vi "StringToVariant.vi"(7 "use system decimal point (T)":bool=TRUE, 11 "String-formatted Value":string) -> (2 "Value Class":T1, 3 "Variant-formatted Value":variant)   [LabVIEW 2013, in "CfgManager.Text.lvlib" / "Serializer.PlainText.lvclass"]
uses:
  Serializer.PlainText.lvclass
  Manager.Text/Character Class -- Enum.ctl
  Manager.Text/ConfigManager.Text.lvclass
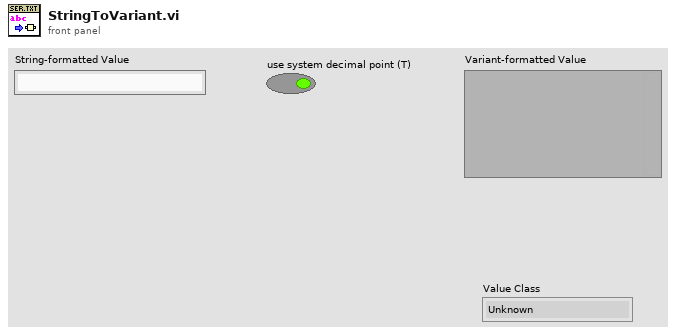
[diagram p1: front panel]
types:
  T1 = typedef "CfgManager.Text.lvlib/ConfigManager.Text.lvclass/Character Class -- Enum.ctl" = enum16{"Unknown", "Sign", "Zero", "Integer", "Float", "Complex", "Scientific", "Engineering", "Hexadecimal", "Binary", "Decimal", "Octal", "Unit", "Invalid", "Timestamp", "Boolean", "String", "Path", "null"}
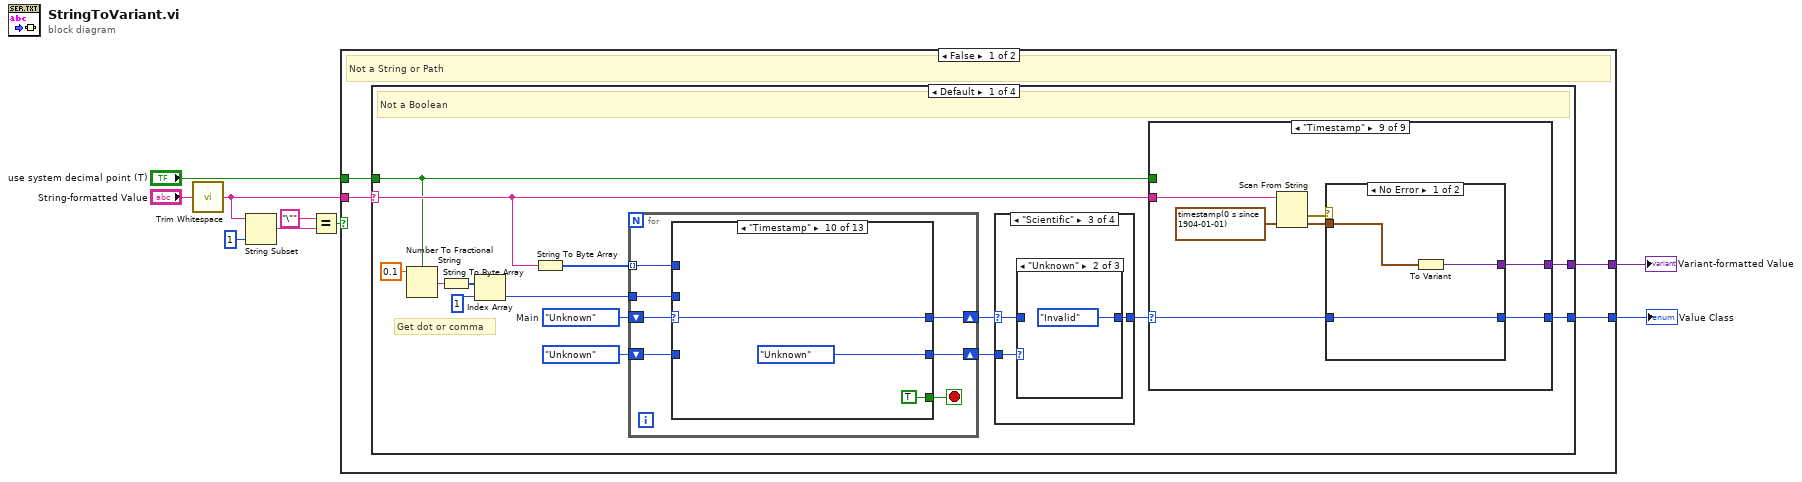
[diagram p0: block diagram]
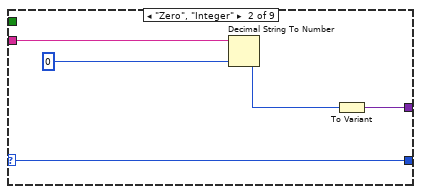
[diagram p3: hidden frame]
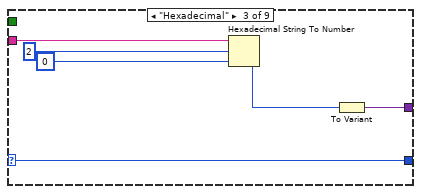
[diagram p4: hidden frame]
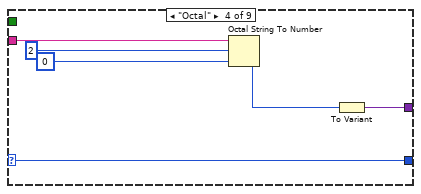
[diagram p5: hidden frame]
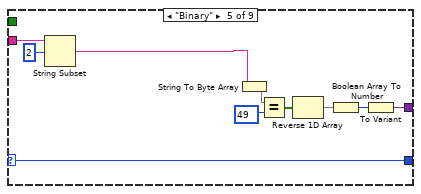
[diagram p6: hidden frame]
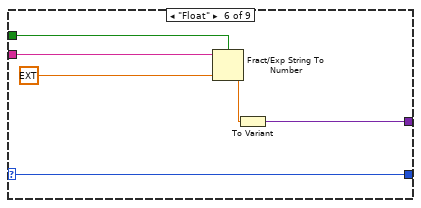
[diagram p7: hidden frame]
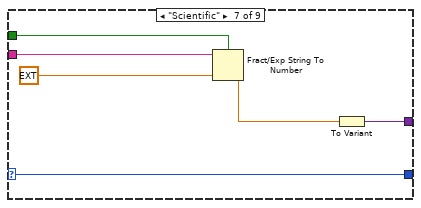
[diagram p8: hidden frame]
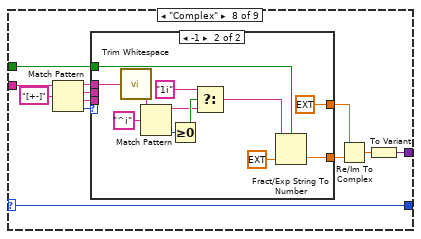
[diagram p9: hidden frame]
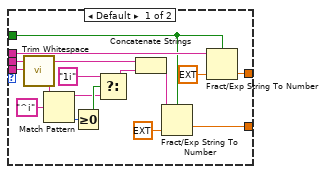
[diagram p10: hidden frame]
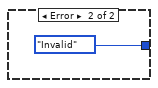
[diagram p11: hidden frame]
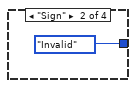
[diagram p13: hidden frame]
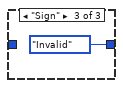
[diagram p15: hidden frame]
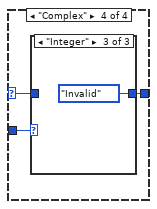
[diagram p16: hidden frame]
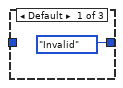
[diagram p17: hidden frame]
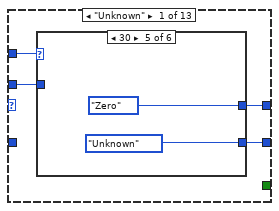
[diagram p19: hidden frame]
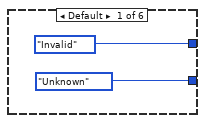
[diagram p20: hidden frame]
diagram:
  n1 = call <vilib>:"Trim Whitespace.vi"("string"="String-formatted Value") -> ("trimmed string"=w8:string)  [unwired: 1 in]
  n2 = String Subset(string=w8, length (rest)=1 ("length (rest)")) -> (substring=w6:string)  [unwired: 1 in]
  n3 = Equal?(x="\"", y=w6) -> (x = y?=w4:bool)
  n4 = case shown="False" w4 {
    tunnel: w8 -> [w13 w387]
    tunnel: [w12 w390] -> w9
    tunnel: [w11 w382] -> w3
    tunnel: "use system decimal point (T)" -> [w10 _]
    frame False {
      # "Not a String or Path"
      n5 = case shown="Default" w13 {
        selector: w13 -> [w23 _ _ _]
        tunnel: [w22 w374 w377 w381] -> w12
        tunnel: [w21 Character_Class_--_Enum."Boolean" Character_Class_--_Enum."Boolean" Character_Class_--_Enum."null"] -> w11
        tunnel: w10 -> [w18 _ _ _]
        frame Default {
          w27 = Character_Class_--_Enum."Unknown"  # Main
          # "Get dot or comma"
          # "Not a Boolean"
          n6 = Number To Fractional String(use system decimal point (T)=w18, number=0.1) -> (F-format string=w16:string)  [unwired: 2 in]
          n7 = String To Byte Array(string=w16) -> (unsigned byte array=w17:u8[])
          n8 = Index Array(array=w17, index=1 ("length (rest)")) -> (element=w14:u8)
          n9 = String To Byte Array(string=w23) -> (unsigned byte array=w28:u8[])
          n10 = for {
            tunnel: w28 -> [w139] mode=indexing
            shift-right: [w138] -> w26
            shift-left: w27 -> [w140]
            shift-right: [w136] -> w25
            shift-left: Character_Class_--_Enum."Unknown" -> [w137]
            tunnel: w14 -> [w134]
            stop <- w135 stop-if-true
            n11 = case shown="\"Timestamp\"" w140 {
              selector: w140 -> [_ w163 w167 w186 w217 w240 w246 w252 w258 w264 w267 w283 w324]
              tunnel: w139 -> [w144 _ w169 w188 w219 w242 w248 w254 w260 _ w269 w285 w326]
              tunnel: [w143 w163 w168 w187 w218 w241 w247 w253 w259 w264 w268 w284 w325] -> w138
              tunnel: w137 -> [_ w162 w164 _ _ _ _ _ _ _ _ w282 w323]
              tunnel: [w142 w162 w165 w185 w216 Character_Class_--_Enum."Unknown" Character_Class_--_Enum."Unknown" Character_Class_--_Enum."Unknown" Character_Class_--_Enum."Unknown" Character_Class_--_Enum."Unknown" w266 w281 w322] -> w136
              tunnel: [_ TRUE _ _ _ _ _ _ _ TRUE _ _ _] -> w135
              tunnel: w134 -> [w141 _ w166 w184 w215 _ _ _ _ _ _ _ w321]
              frame "Unknown" {
                n12 = case shown="30" w144 {
                  selector: w144 -> [_ _ _ w155 _ _]
                  tunnel: [Character_Class_--_Enum."Invalid" Character_Class_--_Enum."Sign" Character_Class_--_Enum."Integer" w151 Character_Class_--_Enum."Zero" w160] -> w143
                  tunnel: [Character_Class_--_Enum."Unknown" Character_Class_--_Enum."Unknown" Character_Class_--_Enum."Unknown" Character_Class_--_Enum."Unknown" Character_Class_--_Enum."Unknown" w160] -> w142
                  tunnel: w141 -> [_ _ _ w156 _ _]
                  frame Default {
                  }
                  frame 43, 45 {
                  }
                  frame 49..57 {
                  }
                  frame 44, 46 {
                    n13 = Equal?(x=w155, y=w156) -> (x = y?=w154:bool)
                    n14 = Select(t=Character_Class_--_Enum."Float", s=w154, f=Character_Class_--_Enum."Invalid") -> (s? t:f=w151:T1)
                  }
                  frame 48 {
                  }
                  frame 105 {
                    w160 = Character_Class_--_Enum."Complex"
                  }
                }
              }
              frame "Invalid", Default {
              }
              frame "Sign" {
                n15 = case shown="69" w169 {
                  selector: w169 -> [_ _ _ _ w180]
                  tunnel: [Character_Class_--_Enum."Invalid" w173 Character_Class_--_Enum."Integer" w176 w178] -> w168
                  tunnel: w167 -> [_ w173 _ _ _]
                  tunnel: w166 -> [_ _ _ _ w179]
                  tunnel: [Character_Class_--_Enum."Unknown" w172 Character_Class_--_Enum."Unknown" w176 Character_Class_--_Enum."Unknown"] -> w165
                  tunnel: w164 -> [_ w172 _ _ _]
                  frame Default {
                  }
                  frame 32 {
                    # "space (ignore)"
                  }
                  frame 48..57 {
                  }
                  frame 105 {
                    w176 = Character_Class_--_Enum."Complex"
                  }
                  frame 44, 46 {
                    n16 = Equal?(x=w180, y=w179) -> (x = y?=w183:bool)
                    n17 = Select(t=Character_Class_--_Enum."Float", s=w183, f=Character_Class_--_Enum."Invalid") -> (s? t:f=w178:T1)
                  }
                }
              }
              frame "Zero" {
                n18 = case shown="2C, 2E" w188 {
                  selector: w188 -> [_ _ _ w196 _ _ _ _ _ _ _]
                  tunnel: [Character_Class_--_Enum."Invalid" Character_Class_--_Enum."Integer" w194 w195 Character_Class_--_Enum."Hexadecimal" Character_Class_--_Enum."Binary" Character_Class_--_Enum."Octal" Character_Class_--_Enum."Decimal" w211 w212 Character_Class_--_Enum."Complex"] -> w187
                  tunnel: w186 -> [_ _ w194 _ _ _ _ _ w211 _ _]
                  tunnel: [Character_Class_--_Enum."Unknown" Character_Class_--_Enum."Unknown" Character_Class_--_Enum."Unknown" Character_Class_--_Enum."Unknown" Character_Class_--_Enum."Unknown" Character_Class_--_Enum."Unknown" Character_Class_--_Enum."Unknown" Character_Class_--_Enum."Unknown" Character_Class_--_Enum."Unknown" w212 Character_Class_--_Enum."Unknown"] -> w185
                  tunnel: w184 -> [_ _ _ w197 _ _ _ _ _ _ _]
                  frame Default {
                  }
                  frame 49..57 {
                  }
                  frame 48 {
                  }
                  frame 44, 46 {
                    n19 = Equal?(x=w196, y=w197) -> (x = y?=w200:bool)
                    n20 = Select(t=Character_Class_--_Enum."Float", s=w200, f=Character_Class_--_Enum."Invalid") -> (s? t:f=w195:T1)
                  }
                  frame 120 {
                  }
                  frame 98 {
                  }
                  frame 111 {
                  }
                  frame 100 {
                  }
                  frame 32 {
                  }
                  frame 105 {
                    w212 = Character_Class_--_Enum."Complex"
                  }
                  frame 43, 45 {
                  }
                }
              }
              frame "Integer" {
                n21 = case shown="3A" w219 {
                  selector: w219 -> [_ _ _ _ _ w230 _ _]
                  tunnel: [Character_Class_--_Enum."Invalid" w222 w223 w225 w227 w228 Character_Class_--_Enum."Complex" Character_Class_--_Enum."Scientific"] -> w218
                  tunnel: w217 -> [_ _ _ w225 w227 _ _ _]
                  tunnel: [Character_Class_--_Enum."Unknown" w222 w223 Character_Class_--_Enum."Unknown" Character_Class_--_Enum."Unknown" Character_Class_--_Enum."Unknown" Character_Class_--_Enum."Unknown" Character_Class_--_Enum."Unknown"] -> w216
                  tunnel: w215 -> [_ _ _ _ _ w229 _ _]
                  frame Default {
                  }
                  frame 105 {
                    w222 = Character_Class_--_Enum."Complex"
                  }
                  frame 58 {
                    w223 = Character_Class_--_Enum."Timestamp"
                  }
                  frame 32 {
                  }
                  frame 48..57 {
                  }
                  frame 44, 46 {
                    n22 = Equal?(x=w230, y=w229) -> (x = y?=w233:bool)
                    n23 = Select(t=Character_Class_--_Enum."Float", s=w233, f=Character_Class_--_Enum."Invalid") -> (s? t:f=w228:T1)
                  }
                  frame 43, 45 {
                  }
                  frame 69, 101 {
                  }
                }
              }
              frame "Hexadecimal" {
                n24 = case shown="30..39, 41..46" w242 {
                  tunnel: [Character_Class_--_Enum."Invalid" w244] -> w241
                  tunnel: w240 -> [_ w244]
                  frame Default {
                  }
                  frame 48..57, 65..70 {
                  }
                }
              }
              frame "Decimal" {
                n25 = case shown="30..39" w248 {
                  tunnel: [Character_Class_--_Enum."Invalid" w250] -> w247
                  tunnel: w246 -> [_ w250]
                  frame Default {
                  }
                  frame 48..57 {
                  }
                }
              }
              frame "Octal" {
                n26 = case shown="30..37" w254 {
                  tunnel: [Character_Class_--_Enum."Invalid" w256] -> w253
                  tunnel: w252 -> [_ w256]
                  frame Default {
                  }
                  frame 48..55 {
                  }
                }
              }
              frame "Binary" {
                n27 = case shown="30, 31" w260 {
                  tunnel: [Character_Class_--_Enum."Invalid" w262] -> w259
                  tunnel: w258 -> [_ w262]
                  frame Default {
                  }
                  frame 48, 49 {
                  }
                }
              }
              frame "Timestamp" {
              }
              frame "Float" {
                n28 = case shown="2B, 2D" w269 {
                  tunnel: [Character_Class_--_Enum."Invalid" w273 Character_Class_--_Enum."Scientific" w277 Character_Class_--_Enum."Complex" w280] -> w268
                  tunnel: w267 -> [_ w273 _ w277 _ _]
                  tunnel: [Character_Class_--_Enum."Unknown" Character_Class_--_Enum."Unknown" Character_Class_--_Enum."Unknown" Character_Class_--_Enum."Unknown" Character_Class_--_Enum."Unknown" w280] -> w266
                  frame Default {
                  }
                  frame 48..57 {
                  }
                  frame 69, 101 {
                  }
                  frame 32 {
                  }
                  frame 43, 45 {
                  }
                  frame 105 {
                    w280 = Character_Class_--_Enum."Complex"
                  }
                }
              }
              frame "Scientific" {
                n29 = case shown="2B, 2D" w285 {
                  tunnel: [Character_Class_--_Enum."Invalid" w289 w301 w314] -> w284
                  tunnel: w283 -> [_ w288 w303 w316]
                  tunnel: w282 -> [w286 w290 w302 w315]
                  tunnel: [w286 w291 w304 w317] -> w281
                  frame Default {
                  }
                  frame 49..57 {
                    n30 = case shown="\"Unknown\"" w290 {
                      selector: w290 -> [_ _ _ w297 _]
                      tunnel: [w292 Character_Class_--_Enum."Integer" Character_Class_--_Enum."Integer" w297 Character_Class_--_Enum."Integer"] -> w291
                      tunnel: [w292 w293 w296 w298 w300] -> w289
                      tunnel: w288 -> [_ w293 w296 w298 w300]
                      frame Default {
                        w292 = Character_Class_--_Enum."Invalid"
                      }
                      frame "Sign" {
                      }
                      frame "Zero" {
                      }
                      frame "Integer" {
                      }
                      frame "Unknown" {
                      }
                    }
                  }
                  frame 48 {
                    n31 = case shown="\"Sign\"" w302 {
                      tunnel: [w305 Character_Class_--_Enum."Zero" Character_Class_--_Enum."Zero" Character_Class_--_Enum."Zero" Character_Class_--_Enum."Integer"] -> w304
                      tunnel: w303 -> [_ w306 w308 w310 w312]
                      tunnel: [w305 w306 w308 w310 w312] -> w301
                      frame Default {
                        w305 = Character_Class_--_Enum."Invalid"
                      }
                      frame "Unknown" {
                      }
                      frame "Sign" {
                      }
                      frame "Zero" {
                      }
                      frame "Integer" {
                      }
                    }
                  }
                  frame 43, 45 {
                    n32 = case shown="\"Unknown\"" w315 {
                      tunnel: [w318 Character_Class_--_Enum."Sign"] -> w317
                      tunnel: w316 -> [_ w319]
                      tunnel: [w318 w319] -> w314
                      frame Default {
                        w318 = Character_Class_--_Enum."Invalid"
                      }
                      frame "Unknown" {
                      }
                    }
                  }
                }
              }
              frame "Complex" {
                n33 = case shown="2C, 2E" w326 {
                  selector: w326 -> [_ _ _ w342 _]
                  tunnel: [w327 w329 w332 w345 w364] -> w325
                  tunnel: w324 -> [_ w329 w330 w343 w362]
                  tunnel: w323 -> [_ w328 w333 w346 w365]
                  tunnel: [w327 w328 w331 w344 w363] -> w322
                  tunnel: w321 -> [_ _ _ w341 _]
                  frame Default {
                    w327 = Character_Class_--_Enum."Invalid"
                  }
                  frame 32 {
                  }
                  frame 48..57 {
                    n34 = case shown="Default" w333 {
                      selector: w333 -> [_ _ w337 w339]
                      tunnel: [w334 w336 w338 w340] -> w332
                      tunnel: [w334 Character_Class_--_Enum."Integer" w337 w339] -> w331
                      tunnel: w330 -> [_ w336 w338 w340]
                      frame Default {
                        w334 = Character_Class_--_Enum."Invalid"
                      }
                      frame "Unknown" {
                      }
                      frame "Integer" {
                      }
                      frame "Float" {
                      }
                    }
                  }
                  frame 44, 46 {
                    n35 = case shown="\"Unknown\"" w346 {
                      tunnel: [w347 w354 w361] -> w345
                      tunnel: [w347 w348 w357] -> w344
                      tunnel: w343 -> [_ w354 w361]
                      tunnel: w342 -> [_ w350 w356]
                      tunnel: w341 -> [_ w349 w355]
                      frame Default {
                        w347 = Character_Class_--_Enum."Invalid"
                      }
                      frame "Unknown" {
                        n36 = Equal?(x=w350, y=w349) -> (x = y?=w353:bool)
                        n37 = Select(t=Character_Class_--_Enum."Float", s=w353, f=Character_Class_--_Enum."Invalid") -> (s? t:f=w348:T1)
                      }
                      frame "Integer" {
                        n38 = Equal?(x=w356, y=w355) -> (x = y?=w360:bool)
                        n39 = Select(t=Character_Class_--_Enum."Float", s=w360, f=Character_Class_--_Enum."Invalid") -> (s? t:f=w357:T1)
                      }
                    }
                  }
                  frame 105 {
                    n40 = case shown="\"Float\"" w365 {
                      tunnel: [w366 w368 w370 w372] -> w364
                      tunnel: [w366 Character_Class_--_Enum."Complex" Character_Class_--_Enum."Complex" Character_Class_--_Enum."Complex"] -> w363
                      tunnel: w362 -> [_ w368 w370 w372]
                      frame Default {
                        w366 = Character_Class_--_Enum."Invalid"
                      }
                      frame "Unknown" {
                      }
                      frame "Integer" {
                      }
                      frame "Float" {
                      }
                    }
                  }
                }
              }
            }
          }
          n41 = case shown="\"Scientific\"" w26 {
            selector: w26 -> [w120 _ w122 w128]
            tunnel: w25 -> [_ _ w124 w130]
            tunnel: [w120 Character_Class_--_Enum."Invalid" w123 w129] -> w24
            frame Default {
            }
            frame "Sign" {
            }
            frame "Scientific" {
              n42 = case shown="\"Unknown\"" w124 {
                tunnel: [w125 Character_Class_--_Enum."Invalid" Character_Class_--_Enum."Invalid"] -> w123
                tunnel: w122 -> [w125 _ _]
                frame Default {
                }
                frame "Unknown" {
                }
                frame "Sign" {
                }
              }
            }
            frame "Complex" {
              n43 = case shown="\"Integer\"" w130 {
                tunnel: [Character_Class_--_Enum."Invalid" w132 Character_Class_--_Enum."Invalid" ("Main")] -> w129
                tunnel: w128 -> [_ w132 _]
                frame Default {
                }
                frame "Complex" {
                }
                frame "Integer" {
                }
              }
            }
          }
          n44 = case shown="\"Timestamp\"" w24 {
            selector: w24 -> [w29 w30 w35 w41 w47 w58 w64 w79 w109]
            tunnel: w23 -> [_ w34 w40 w46 w55 w62 w68 w75 w115]
            tunnel: [_ w31 w37 w43 w56 w59 w65 w80 w112] -> w22
            tunnel: [w29 w30 w35 w41 w47 w58 w64 w79 w110] -> w21
            tunnel: w18 -> [_ _ _ _ _ w57 w63 w70 _]
            frame Default {
            }
            frame "Zero", "Integer" {
              n45 = Decimal String To Number(string=w34, default (0L)=i64 0 ("default (0 I32)")) -> (number=w32:i64)  [unwired: 1 in, 1 out]
              n46 = To Variant(anything=w32) -> (Variant=w31:variant)
            }
            frame "Hexadecimal" {
              n47 = Hexadecimal String To Number(string=w40, offset=2, default (0uL)=i64 0 ("default (0 I32)")) -> (number=w38:i64)  [unwired: 1 out]
              n48 = To Variant(anything=w38) -> (Variant=w37:variant)
            }
            frame "Octal" {
              n49 = Octal String To Number(2:i64 0 ("default (0 I32)"), 3:2 ("offset"), 4:w46) -> (0:w44:i64)  [unwired: 1 out]
              n50 = To Variant(anything=w44) -> (Variant=w43:variant)
            }
            frame "Binary" {
              n51 = String Subset(string=w55, offset (0)=2) -> (substring=w53:string)  [unwired: 1 in]
              n52 = String To Byte Array(string=w53) -> (unsigned byte array=w51:u8[])
              n53 = Equal?(x=w51, y=u8 49 ("offset (0)")) -> (x = y?=w50:bool[])
              n54 = Reverse 1D Array(array=w50) -> (reversed array=w48:bool[])
              n55 = Boolean Array To Number(Boolean array=w48) -> (number=w52:u32)
              n56 = To Variant(anything=w52) -> (Variant=w56:variant)
            }
            frame "Float" {
              n57 = Fract/Exp String To Number(use system decimal point (T)=w57, string=w62, default (0 dbl)=ext 0.0 ("default (0 I32)")) -> (number=w60:ext)  [unwired: 1 in, 1 out]
              n58 = To Variant(anything=w60) -> (Variant=w59:variant)
            }
            frame "Scientific" {
              n59 = Fract/Exp String To Number(use system decimal point (T)=w63, string=w68, default (0 dbl)=ext 0.0 ("default (0 I32)")) -> (number=w66:ext)  [unwired: 1 in, 1 out]
              n60 = To Variant(anything=w66) -> (Variant=w65:variant)
            }
            frame "Complex" {
              n61 = Match Pattern(string=w75, regular expression="[+-]") -> (before substring=w72:string, match substring=w69:string, after substring=w71:string, offset past match=w76:i32)  [unwired: 1 in]
              n62 = case shown="-1" w76 {
                tunnel: [w93 ext 0.0 ("default (0 DBL)")] -> w73
                tunnel: [w95 w106] -> w74
                tunnel: w72 -> [w92 w98]
                tunnel: w71 -> [w82 _]
                tunnel: w70 -> [w91 w105]
                tunnel: w69 -> [w85 _]
                frame Default {
                  n63 = call <vilib>:"Trim Whitespace.vi"("string"=w82) -> ("trimmed string"=w83:string)  [unwired: 1 in]
                  n64 = Match Pattern(string=w83, regular expression="^i") -> (before substring=w88:string, offset past match=w90:i32)  [unwired: 1 in, 2 out]
                  n65 = Greater Or Equal To 0?(x=w90) -> (x >= 0?=w89:bool)
                  n66 = Select(t="1i", s=w89, f=w88) -> (s? t:f=w86:string)
                  n67 = Concatenate Strings(w85, w86) -> (w84:string)
                  n68 = Fract/Exp String To Number(use system decimal point (T)=w91, string=w84, default (0 dbl)=ext 0.0 ("default (0 DBL)")) -> (number=w95:ext)  [unwired: 1 in, 1 out]
                  n69 = Fract/Exp String To Number(use system decimal point (T)=w91, string=w92, default (0 dbl)=ext 0.0 ("default (0 DBL)")) -> (number=w93:ext)  [unwired: 1 in, 1 out]
                }
                frame -1 {
                  n70 = call <vilib>:"Trim Whitespace.vi"("string"=w98) -> ("trimmed string"=w100:string)  [unwired: 1 in]
                  n71 = Match Pattern(string=w100, regular expression="^i") -> (before substring=w102:string, offset past match=w104:i32)  [unwired: 1 in, 2 out]
                  n72 = Greater Or Equal To 0?(x=w104) -> (x >= 0?=w103:bool)
                  n73 = Select(t="1i", s=w103, f=w102) -> (s? t:f=w97:string)
                  n74 = Fract/Exp String To Number(use system decimal point (T)=w105, string=w97, default (0 dbl)=ext 0.0 ("default (0 DBL)")) -> (number=w106:ext)  [unwired: 1 in, 1 out]
                }
              }
              n75 = Re/Im To Complex(1:w74, 2:w73) -> (0:w78:cxt)
              n76 = To Variant(anything=w78) -> (Variant=w80:variant)
            }
            frame "Timestamp" {
              n77 = Scan From String(input string=w115, default 1=timestamp(0 s since 1904-01-01)) -> (error out=w111:errorcluster, output 1=w113:timestamp)  [unwired: 3 in, 2 out]
              n78 = case shown="No Error" w111 {
                tunnel: w113 -> [w118 _]
                tunnel: [w117 _] -> w112
                tunnel: [w116 Character_Class_--_Enum."Invalid"] -> w110
                tunnel: w109 -> [w116 _]
                frame No Error {
                  n79 = To Variant(anything=w118) -> (Variant=w117:variant)
                }
                frame Error {
                }
              }
            }
          }
        }
        frame "true" {
          # "BOOLEAN (TRUE)"
          n80 = To Variant(anything=TRUE) -> (Variant=w374:variant)
        }
        frame "false" {
          # "BOOLEAN (FALSE)"
          n81 = To Variant(anything=FALSE) -> (Variant=w377:variant)
        }
        frame "null" {
          # "null"
          n82 = To Variant(anything=variant ("variant")) -> (Variant=w381:variant)
        }
      }
    }
    frame True {
      # "String or Path"
      n83 = String Length(string=w387) -> (length=w389:i32)
      n84 = Decrement(x=w389) -> (x-1=w384:i32)
      n85 = String Subset(string=w387, offset (0)=w384, length (rest)=1 ("length (rest)")) -> (substring=w385:string)
      n86 = Equal?(x=w385, y="\"" ("x")) -> (x = y?=w383:bool)
      n87 = case shown="True" w383 {
        tunnel: [_ w393] -> w390
        tunnel: w387 -> [_ w404]
        tunnel: w384 -> [_ w403]
        tunnel: [Character_Class_--_Enum."Invalid" w392] -> w382
        frame False {
        }
        frame True {
          n88 = Decrement(x=w403) -> (x-1=w402:i32)
          n89 = String Subset(string=w404, offset (0)=1, length (rest)=w402) -> (substring=w394:string)
          n90 = String Subset(string=w394, length (rest)=1 ("length (rest)")) -> (substring=w400:string)  [unwired: 1 in]
          n91 = Equal?(x="/", y=w400) -> (x = y?=w398:bool)
          n92 = Select(t=u8 50 ("Type"), s=w398, f=u8 48 ("Type")) -> (s? t:f=w395:u8)
          n93 = case shown="32" w395 {
            tunnel: [w409 w412] -> w393
            tunnel: w394 -> [w408 w410]
            tunnel: [Character_Class_--_Enum."Path" Character_Class_--_Enum."String"] -> w392
            frame 50 {
              # "PATH (0x32)"
              n94 = call "Common Path to Specific Path.vi"("common path"=w408) -> ("specific path"=w407:path)  [unwired: 10 in]
              n95 = To Variant(anything=w407) -> (Variant=w409:variant)
            }
            frame 48, Default {
              # "STRING (0x30)"
              n96 = To Variant(anything=w410) -> (Variant=w412:variant)
            }
          }
        }
      }
    }
  }
  "Variant-formatted Value" <- w9
  "Value Class" <- w3
